vi "Get Signing Error String.vi"(8 "error in (no error)":errorcluster, 11 "NICSGN_ERROR":i64) -> (0 "error out":errorcluster)   [LabVIEW 2020, in "CodeSignAPI.lvlib"]
doc: "GetSigningErrorString(NICSGN_ERROR err, char * buff);"
uses:
  <vilib>/AppBuilder/CodeSignAPI/CodeSignAPI.lvlib
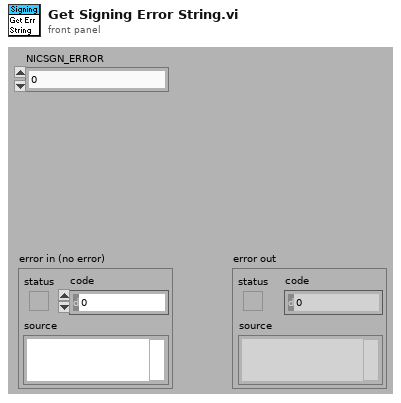
[diagram p1: front panel]
types:
  T1 = typedef "sTypeDef_Languages.ctl" = u16
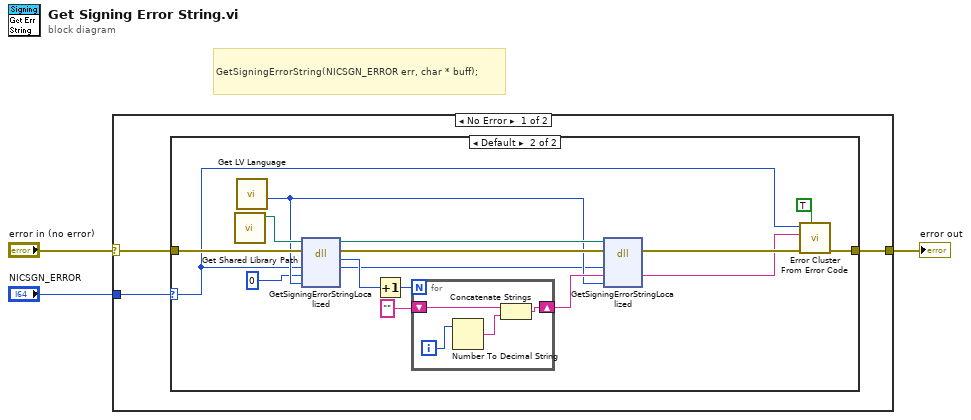
[diagram p0: block diagram]
diagram:
  # "GetSigningErrorString(NICSGN_ERROR err, char * buff);"
  n1 = case shown="No Error" "error in (no error)" {
    selector: "error in (no error)" -> [w5 w28]
    tunnel: "NICSGN_ERROR" -> [w4 _]
    tunnel: [w6 w28] -> w2
    frame No Error {
      n2 = case shown="Default" w4 {
        selector: w4 -> [_ w8]
        tunnel: [w7 w23] -> w6
        tunnel: w5 -> [w7 w21]
        frame 0.. {
        }
        frame Default {
          n3 = call <vilib>:"Get Shared Library Path.vi"() -> ("shared library path"=w22:path)  [unwired: 1 in, 10 out]
          n4 = call <vilib>:"Get LV Language.vi"() -> ("Language"=w11:T1)  [unwired: 11 out]
          n5 = dll-call lib="?" fn="GetSigningErrorStringLocalized"(path in=w22, error in=w21, "err"=w8, "buff"=u64 0, "languageID"=w11) -> (path out=w16:path, error out=w19:errorcluster, "return type"=w13:i32, "err"=w10:i64)  [unwired: 1 in, 2 out]
          n6 = Increment(x=w13) -> (x+1=w14:i32)
          n7 = for {
            N: w14 -> [_]
            shift-right: [w24] -> w12
            shift-left: "" -> [w25]
            i -> [w27]
            n8 = Number To Decimal String(number=w27) -> (decimal integer string=w26:string)  [unwired: 1 out]
            n9 = Concatenate Strings(w25, w26) -> (w24:string)
          }
          n10 = dll-call lib="?" fn="GetSigningErrorStringLocalized"(path in=w16, error in=w19, "err"=w10, "buff"=w12, "languageID"=w11) -> (error out=w18:errorcluster, "buff"=w17:string)  [unwired: 2 in, 3 out]
          n11 = call <vilib>:"Error Cluster From Error Code.vi"("show call chain? (False)"=TRUE, "error in (no error)"=w18, "error message (\"\")"=w17, "error code (0)"=w8) -> ("error out"=w23:errorcluster)  [unwired: 5 out]
        }
      }
    }
    frame Error {
    }
  }
  "error out" <- w2
